vi "IIOA_mxwQueryRegSystemString.vi"(8 "error in (no error)":errorcluster, 10 "valueName":string="Path", 11 "KeyName":string="Software\\National Instruments\\Assistants") -> (0 "error out":errorcluster, 3 "Result":string)   [LabVIEW 2019]
uses:
  <vilib>/registry/registry.llb/Registry SAM.ctl
  <vilib>/registry/registry.llb/Read Registry Value Simple STR.vi
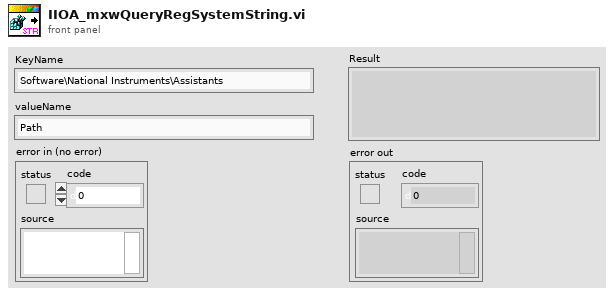
[diagram p1: front panel]
types:
  T1 = typedef "Registry SAM.ctl" = enum32{"KEY_QUERY_VALUE", "KEY_SET_VALUE", "KEY_CREATE_SUB_KEY", "KEY_ENUMERATE_SUB_KEYS", "KEY_NOTIFY", "KEY_CREATE_LINK", "KEY_READ", "KEY_WRITE", "KEY_ALL_ACCESS", "KEY_READ | KEY_WRITE"}
  T2 = typedef "Registry refnum.ctl" = refnum<k1>
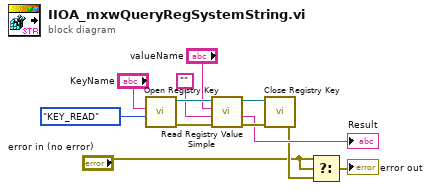
[diagram p0: block diagram]
diagram:
  n1 = call <vilib>:"Open Registry Key.vi"("security access mask (KEY_READ | KEY_WRITE)"=Registry_SAM."KEY_READ", "subkey"="KeyName") -> ("error out"=w12:errorcluster, "refnum out"=w11:T2)  [unwired: 8 in]
  n2 = call-poly <vilib>:"Read Registry Value Simple.vi"("error in (no error)"=w12, "default data"="", "value"="valueName", "refnum"=w11) -> ("error out"=w8:errorcluster, "String/Binary data"=→"Result":string, "refnum out"=w9:T2)  [unwired: 2 in, 1 out]
  n3 = call <vilib>:"Close Registry Key.vi"("error in (no error)"=w8, "refnum"=w9) -> ("error out"=w5:errorcluster)  [unwired: 5 in]
  n4 = Select(t="error in (no error)", s="error in (no error)", f=w5) -> (s? t:f=→"error out":errorcluster)
